vi "Click Callback.vi"(4 "onClick":refnum<user-event>, 5 "Event Data":cluster{"sender":refnum<k24>, "e":refnum<k24>}, 6 "Control Ref":refnum<k24>, 7 "Event Common Data":T1) -> ()   [LabVIEW 2024, in "SourceGrid.lvlib" / "Custom Events.lvclass"]
uses:
  Custom Events.lvclass
  D:/git/Sourcegrid-LabVIEW/dll/SourceGrid.dll
  dll/SourceGrid.dll
  Cells/Cell Context/Cell Context.lvclass
  Custom Events.lvclass/Custom Events.ctl
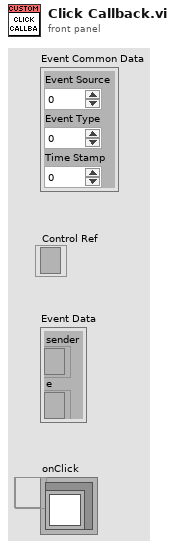
[diagram p1: front panel]
types:
  T1 = cluster{"Event Source":i32, "Event Type":u32, "Time Stamp":u32}
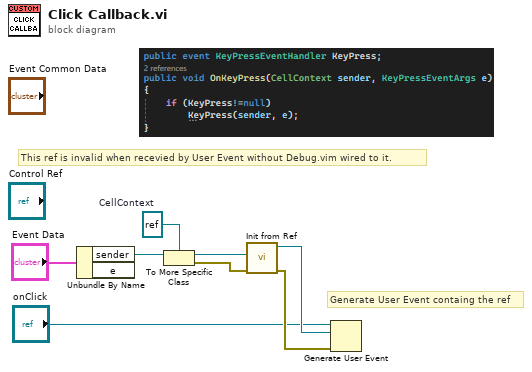
[diagram p0: block diagram]
diagram:
  w6 = refnum<k24> refnum  # CellContext
  # "Generate User Event containg the ref"
  # "This ref is invalid when recevied by User Event without Debug.vim wired to it."
  n1 = Unbundle By Name("Event Data") -> ("sender"=w7:refnum<k24>)  [unwired: 1 out]
  n2 = To More Specific Class(target class=w6, reference=w7) -> (specific class reference=w1:refnum<k24>, error out=w5:errorcluster)  [unwired: 1 in]
  n3 = call "Init from Ref.vi"("error in"=w5, "CellContext .NET"=w1) -> ("error out"=w3:errorcluster, "Cell Context out"=w4:refnum<class "Cell Context.lvclass">)  [unwired: 8 in]
  n4 = Generate User Event(user event="onClick", event data cluster=w4, error in=w3) -> ()  [unwired: 1 in, 2 out]
